vi "Set T.vi"(0 "Set point":dbl format="%.2f", 1 "GPIB Adress":i16) -> ()   [LabVIEW 2015]
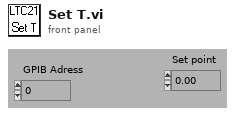
[diagram p1: front panel]
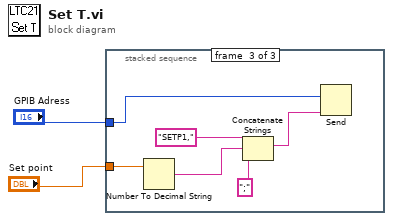
[diagram p0: block diagram]
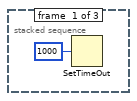
[diagram p2: hidden frame]
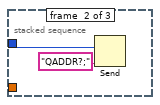
[diagram p3: hidden frame]
diagram:
  n1 = stacked-sequence {
    tunnel: "GPIB Adress" -> [_ w5 w11]
    tunnel: "Set point" -> [_ _ w7]
    frame #0 {
      n2 = SetTimeOut(1:1000 ("new timeout (10000)")) -> ()  [unwired: 1 out]
    }
    frame #1 {
      n3 = Send(2:w5, 5:"QADDR?;" ("data string")) -> ()  [unwired: 3 in, 3 out]
    }
    frame #2 {
      n4 = Number To Decimal String(number=w7) -> (decimal integer string=w9:string)  [unwired: 1 in]
      n5 = Concatenate Strings("SETP1," ("data string"), w9, ";" ("Substring")) -> (w6:string)
      n6 = Send(2:w11, 5:w6) -> ()  [unwired: 3 in, 3 out]
    }
  }
